vi "tsapp_get_hw_info_by_index_verbose.vi"(8 "error in":errorcluster, 10 "AIndex":i32, 11 "路径输入":path) -> (0 "error out":errorcluster, 1 "DeviceName":string, 2 "VendorName":string, 3 "路径输出":path, 4 "Hardware Type":T1=8 items=["BUS_UNKNOWN_TYPE", "TS_TCP_DEVICE", "XL_USB_DEVICE", "TS_USB_DEVICE", "PEAK_USB_DEVICE", "KVASER_USB_DEVICE", "ZLG_USB_DEVICE", "ICS_USB_DEVICE", "TS_TC1005_DEVICE", "CANABLE_USB_DEVICE", "TS_WIRELESS_OBD", "TS_USB_DEVICE_EX", "IXXAT_USB_DEVICE", "TS_ETH_IF_DEVICE", "TS_USB_IF_DEVICE", "BUS_DEV_TYPE_COUNT"], 5 "SerialNum":string)   [LabVIEW 2014]
doc: "Retrieve information about hardware devices based on index values."
uses:
  Typedef/Hardware Type.ctl
panel:
  out "return":i32
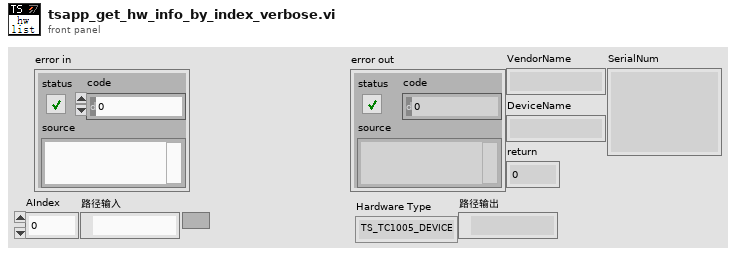
[diagram p1: front panel]
types:
  T1 = typedef "Hardware Type.ctl" = i32
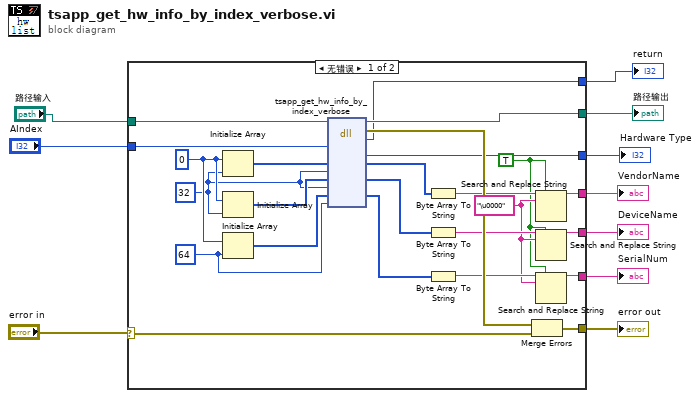
[diagram p0: block diagram]
diagram:
  n1 = case shown="无错误" "error in" {
    selector: "error in" -> [w34 w37]
    tunnel: [w35 w37] -> w10
    tunnel: "AIndex" -> [w32 _]
    tunnel: [w31 _] -> w4
    tunnel: [w20 _] -> w7
    tunnel: [w18 _] -> w6
    tunnel: [w17 _] -> w5
    tunnel: "路径输入" -> [w13 w36]
    tunnel: [w12 w36] -> w2
    tunnel: [w11 _] -> w1
    frame No Error {
      w14 = TRUE ("replace all? (F)")
      w15 = "\u0000" ("substring (\"\")")
      w25 = 64 ("dimension size")
      w26 = 32 ("dimension size")
      w29 = u8 0
      n2 = Initialize Array(w29, w26) -> (w30:u8[])
      n3 = Initialize Array(w29, w26) -> (w28:u8[])
      n4 = Initialize Array(w29, w25) -> (w27:u8[])
      n5 = dll-call lib="D:/Program Files (x86)/TOSUN/TSMaster/bin/TSMaster.dll" fn="tsapp_get_hw_info_by_index_verbose"(path in=w13, "AIndex"=w32, "AVendorNameBuffer"=w30, "AVendorNameBufferSize"=w26, "ADeviceNameBuffer"=w28, "ADeviceNameBufferSize"=w26, "ASerialStringBuffer"=w27, "ASerialStringBufferSize"=w25) -> (path out=w12:path, error out=w33:errorcluster, "result"=w11:i32, "ADeviceType"=w31:i32, "AVendorNameBuffer"=w24:u8[], "ADeviceNameBuffer"=w23:u8[], "ASerialStringBuffer"=w22:u8[])  [unwired: 7 in]
      n6 = Byte Array To String(unsigned byte array=w24) -> (string=w21:string)
      n7 = Byte Array To String(unsigned byte array=w23) -> (string=w19:string)
      n8 = Byte Array To String(unsigned byte array=w22) -> (string=w16:string)
      n9 = Merge Errors(w33, w34) -> (w35:errorcluster)
      n10 = Search and Replace String(replace all?=w14, input string=w21, search string=w15) -> (result string=w20:string)  [unwired: 5 in, 3 out]
      n11 = Search and Replace String(replace all?=w14, input string=w19, search string=w15) -> (result string=w18:string)  [unwired: 5 in, 3 out]
      n12 = Search and Replace String(replace all?=w14, input string=w16, search string=w15) -> (result string=w17:string)  [unwired: 5 in, 3 out]
    }
    frame Error {
    }
  }
  "error out" <- w10
  "VendorName" <- w7
  "DeviceName" <- w6
  "SerialNum" <- w5
  "Hardware Type" <- w4
  "路径输出" <- w2
  "return" <- w1
